vi "NT to Globals & XML.vi"(8 "Array":path[](array[path])) -> ()   [LabVIEW 2020]
uses:
  Utility VIs/NT to XML Number.vi
  Globals/Dashboard_Cal_Globals.vi
panel:
  in  "NT Name Categories":string[](array[string])=["Turret", "Intake", "Magazine", "Flywheel", "FR", "FL", "BL", "BR", "Manual", "Cowl"]
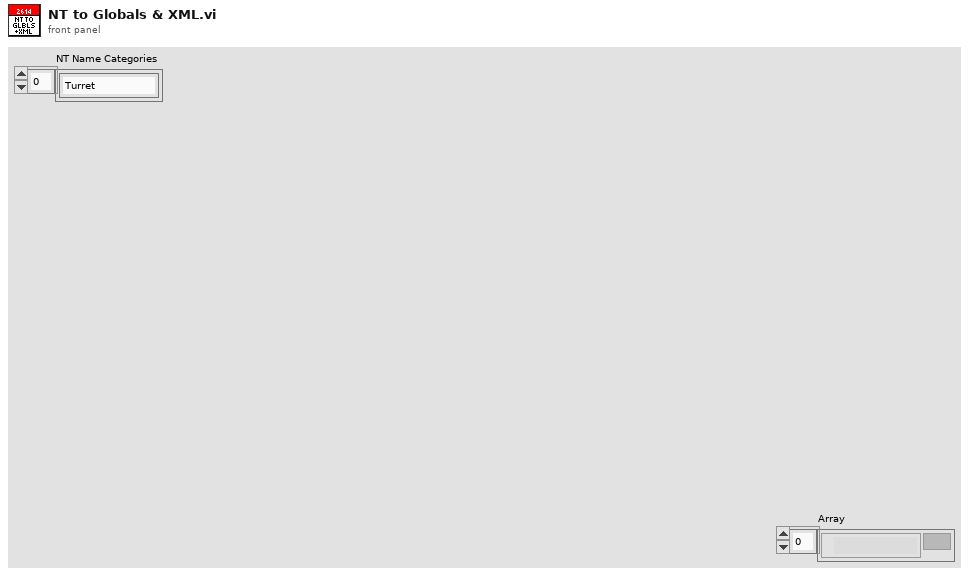
[diagram p1: front panel]
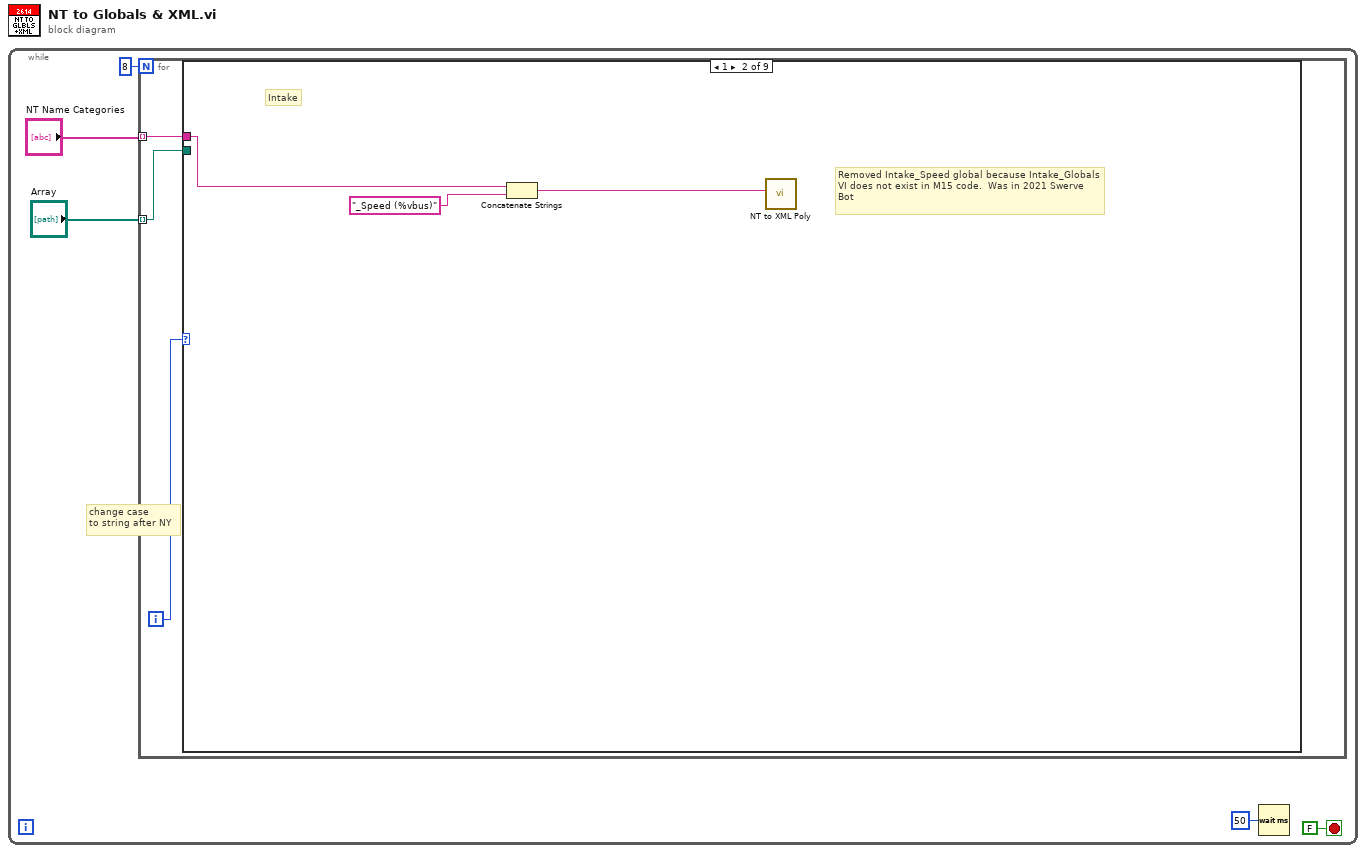
[diagram p0: block diagram]
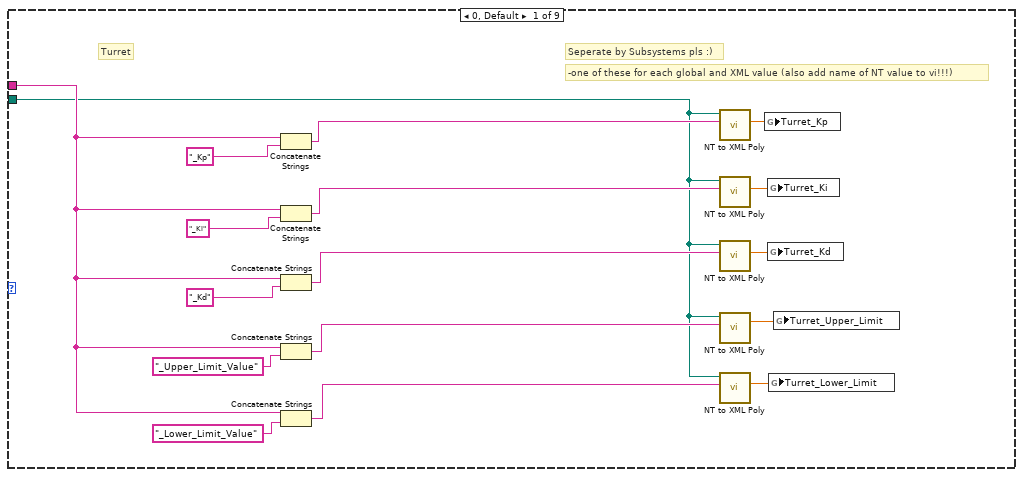
[diagram p2: hidden frame]
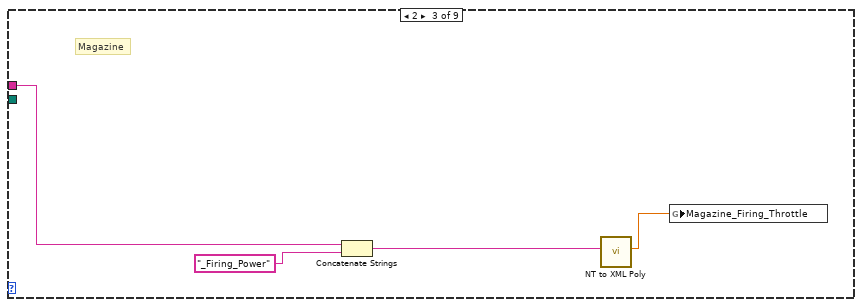
[diagram p3: hidden frame]
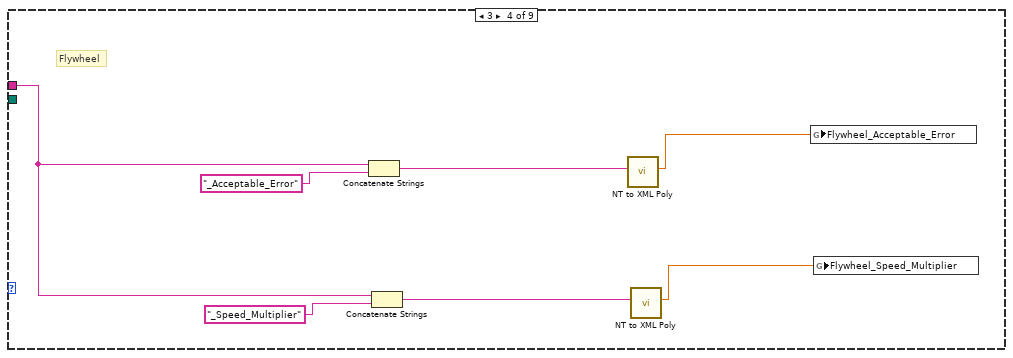
[diagram p4: hidden frame]
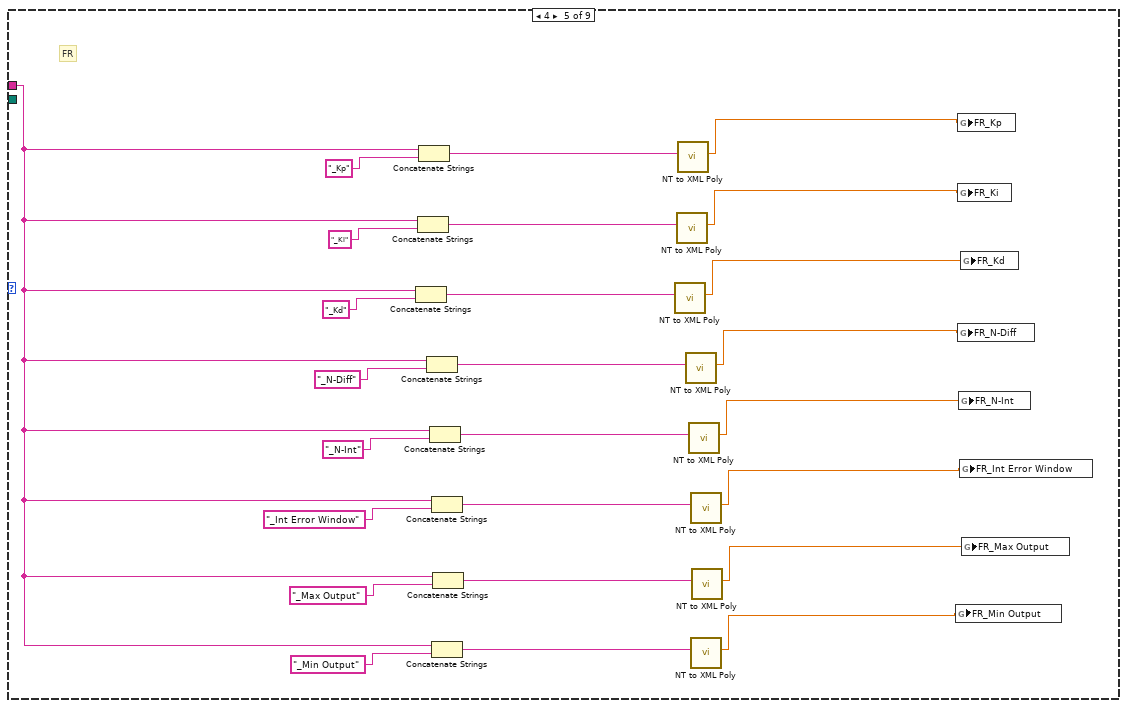
[diagram p5: hidden frame]
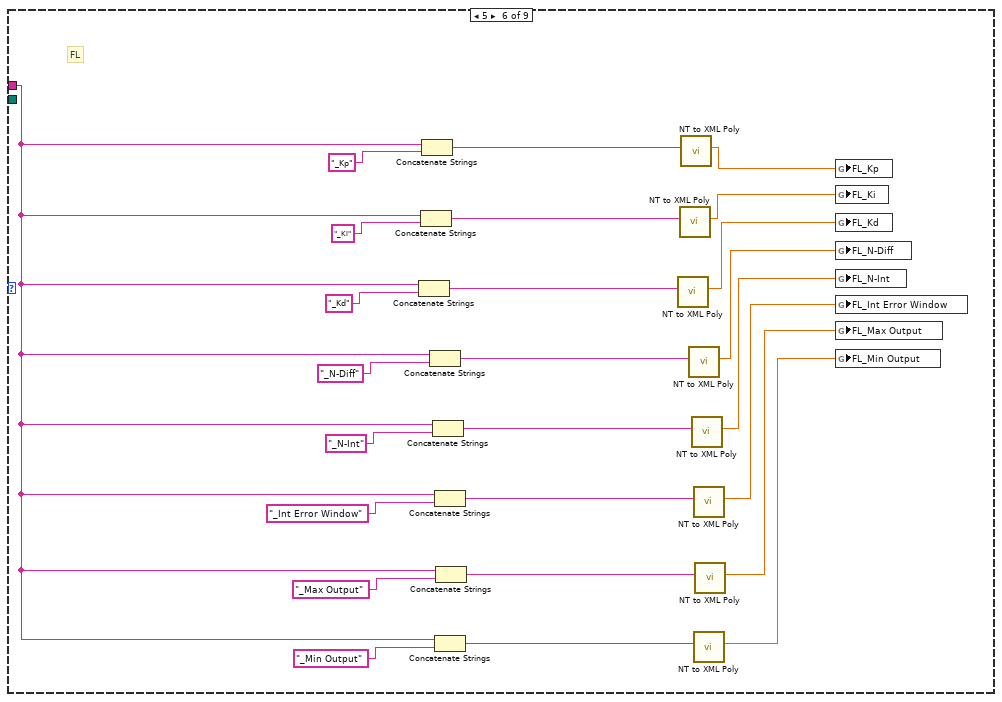
[diagram p6: hidden frame]
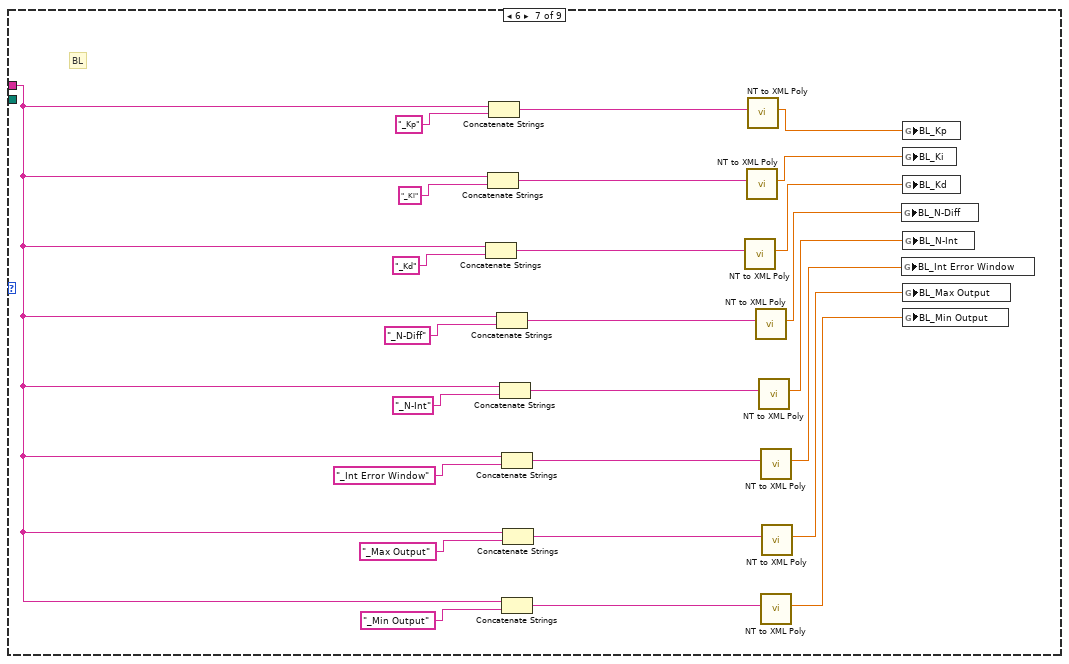
[diagram p7: hidden frame]
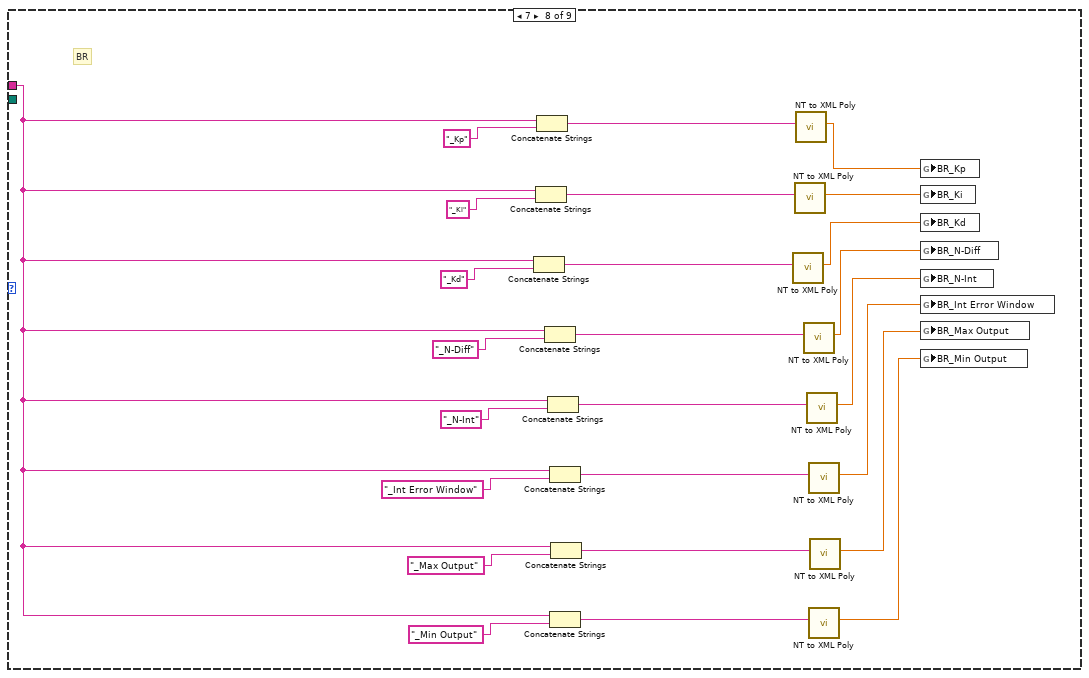
[diagram p8: hidden frame]
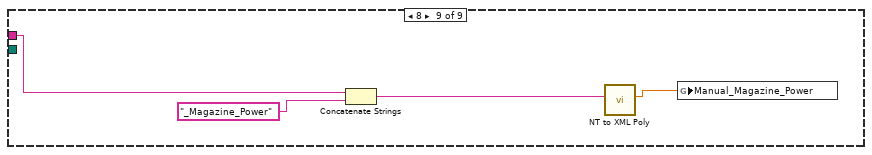
[diagram p9: hidden frame]
diagram:
  n1 = while {
    stop <- FALSE stop-if-true
    # "change case\nto string after NY"
    n2 = for {
      N: 8 -> [_]
      tunnel: "NT Name Categories" -> [w8] mode=indexing
      tunnel: "Array" -> [w7] mode=indexing
      i -> [w6]
      n3 = case shown="1" w6 {
        tunnel: w8 -> [w15 w26 w30 w33 w40 w73 w98 w123 w140]
        tunnel: w7 -> [w9 _ _ _ _ _ _ _ _]
        frame 0, Default {
          # "Turret"
          # "-one of these for each global and XML value (also add name of NT value to vi!!!)"
          # "Seperate by Subsystems pls :)"
          n4 = Concatenate Strings(w15, "_Kp" ("NT Name")) -> (w14:string)
          n5 = Concatenate Strings(w15, "_Ki" ("NT Name")) -> (w13:string)
          n6 = Concatenate Strings(w15, "_Kd" ("NT Name")) -> (w12:string)
          n7 = Concatenate Strings(w15, "_Upper_Limit_Value" ("NT Name")) -> (w11:string)
          n8 = Concatenate Strings(w15, "_Lower_Limit_Value" ("NT Name")) -> (w10:string)
          n9 = call-poly "NT to XML Poly.vi"("NT Name"=w14, "XML File Path"=w9) -> ("Numeric"=w20:dbl)  [unwired: 9 in]
          n10 = call-poly "NT to XML Poly.vi"("NT Name"=w13, "XML File Path"=w9) -> ("Numeric"=w21:dbl)  [unwired: 9 in]
          n11 = call-poly "NT to XML Poly.vi"("NT Name"=w12, "XML File Path"=w9) -> ("Numeric"=w22:dbl)  [unwired: 9 in]
          n12 = call-poly "NT to XML Poly.vi"("NT Name"=w11, "XML File Path"=w9) -> ("Numeric"=w24:dbl)  [unwired: 9 in]
          n13 = call-poly "NT to XML Poly.vi"("NT Name"=w10, "XML File Path"=w9) -> ("Numeric"=w23:dbl)  [unwired: 9 in]
          n14 = global write "Dashboard_Cal_Globals.vi" "Turret_Kp"(w20) -> ()
          n15 = global write "Dashboard_Cal_Globals.vi" "Turret_Ki"(w21) -> ()
          n16 = global write "Dashboard_Cal_Globals.vi" "Turret_Kd"(w22) -> ()
          n17 = global write "Dashboard_Cal_Globals.vi" "Turret_Lower_Limit"(w23) -> ()
          n18 = global write "Dashboard_Cal_Globals.vi" "Turret_Upper_Limit"(w24) -> ()
        }
        frame 1 {
          # "Removed Intake_Speed global because Intake_Globals VI does not exist in M15 code.  Was in 2021 Swerve Bot"
          # "Intake"
          n19 = Concatenate Strings(w26, "_Speed (%vbus)" ("NT Name")) -> (w27:string)
          n20 = call-poly "NT to XML Poly.vi"("NT Name"=w27) -> ()  [unwired: 10 in, 1 out]
        }
        frame 2 {
          # "Magazine"
          n21 = Concatenate Strings(w30, "_Firing_Power" ("NT Name")) -> (w32:string)
          n22 = call-poly "NT to XML Poly.vi"("NT Name"=w32) -> ("Numeric"=w29:dbl)  [unwired: 10 in]
          n23 = global write "Dashboard_Cal_Globals.vi" "Magazine_Firing_Throttle"(w29) -> ()
        }
        frame 3 {
          # "Flywheel"
          n24 = Concatenate Strings(w33, "_Acceptable_Error" ("NT Name")) -> (w39:string)
          n25 = Concatenate Strings(w33, "_Speed_Multiplier" ("NT Name")) -> (w36:string)
          n26 = call-poly "NT to XML Poly.vi"("NT Name"=w39) -> ("Numeric"=w37:dbl)  [unwired: 10 in]
          n27 = call-poly "NT to XML Poly.vi"("NT Name"=w36) -> ("Numeric"=w34:dbl)  [unwired: 10 in]
          n28 = global write "Dashboard_Cal_Globals.vi" "Flywheel_Acceptable_Error"(w37) -> ()
          n29 = global write "Dashboard_Cal_Globals.vi" "Flywheel_Speed_Multiplier"(w34) -> ()
        }
        frame 4 {
          # "FR"
          n30 = Concatenate Strings(w40, "_Kd" ("NT Name")) -> (w60:string)
          n31 = Concatenate Strings(w40, "_Ki" ("NT Name")) -> (w62:string)
          n32 = Concatenate Strings(w40, "_Kp" ("NT Name")) -> (w64:string)
          n33 = Concatenate Strings(w40, "_N-Diff" ("NT Name")) -> (w58:string)
          n34 = Concatenate Strings(w40, "_N-Int" ("NT Name")) -> (w56:string)
          n35 = Concatenate Strings(w40, "_Int Error Window" ("NT Name")) -> (w54:string)
          n36 = Concatenate Strings(w40, "_Min Output" ("NT Name")) -> (w50:string)
          n37 = Concatenate Strings(w40, "_Max Output" ("NT Name")) -> (w52:string)
          n38 = call-poly "NT to XML Poly.vi"("NT Name"=w60) -> ("Numeric"=w46:dbl)  [unwired: 10 in]
          n39 = call-poly "NT to XML Poly.vi"("NT Name"=w62) -> ("Numeric"=w47:dbl)  [unwired: 10 in]
          n40 = call-poly "NT to XML Poly.vi"("NT Name"=w64) -> ("Numeric"=w48:dbl)  [unwired: 10 in]
          n41 = call-poly "NT to XML Poly.vi"("NT Name"=w58) -> ("Numeric"=w45:dbl)  [unwired: 10 in]
          n42 = call-poly "NT to XML Poly.vi"("NT Name"=w56) -> ("Numeric"=w44:dbl)  [unwired: 10 in]
          n43 = call-poly "NT to XML Poly.vi"("NT Name"=w54) -> ("Numeric"=w43:dbl)  [unwired: 10 in]
          n44 = call-poly "NT to XML Poly.vi"("NT Name"=w50) -> ("Numeric"=w41:dbl)  [unwired: 10 in]
          n45 = call-poly "NT to XML Poly.vi"("NT Name"=w52) -> ("Numeric"=w42:dbl)  [unwired: 10 in]
          n46 = global write "Dashboard_Cal_Globals.vi" "FR_Min Output"(w41) -> ()
          n47 = global write "Dashboard_Cal_Globals.vi" "FR_Kp"(w48) -> ()
          n48 = global write "Dashboard_Cal_Globals.vi" "FR_Ki"(w47) -> ()
          n49 = global write "Dashboard_Cal_Globals.vi" "FR_N-Diff"(w45) -> ()
          n50 = global write "Dashboard_Cal_Globals.vi" "FR_N-Int"(w44) -> ()
          n51 = global write "Dashboard_Cal_Globals.vi" "FR_Int Error Window"(w43) -> ()
          n52 = global write "Dashboard_Cal_Globals.vi" "FR_Kd"(w46) -> ()
          n53 = global write "Dashboard_Cal_Globals.vi" "FR_Max Output"(w42) -> ()
        }
        frame 5 {
          # "FL"
          n54 = Concatenate Strings(w73, "_Kd" ("NT Name")) -> (w85:string)
          n55 = Concatenate Strings(w73, "_Ki" ("NT Name")) -> (w87:string)
          n56 = Concatenate Strings(w73, "_Kp" ("NT Name")) -> (w89:string)
          n57 = Concatenate Strings(w73, "_N-Diff" ("NT Name")) -> (w83:string)
          n58 = Concatenate Strings(w73, "_N-Int" ("NT Name")) -> (w81:string)
          n59 = Concatenate Strings(w73, "_Int Error Window" ("NT Name")) -> (w79:string)
          n60 = Concatenate Strings(w73, "_Min Output" ("NT Name")) -> (w75:string)
          n61 = Concatenate Strings(w73, "_Max Output" ("NT Name")) -> (w77:string)
          n62 = call-poly "NT to XML Poly.vi"("NT Name"=w85) -> ("Numeric"=w70:dbl)  [unwired: 10 in]
          n63 = call-poly "NT to XML Poly.vi"("NT Name"=w87) -> ("Numeric"=w71:dbl)  [unwired: 10 in]
          n64 = call-poly "NT to XML Poly.vi"("NT Name"=w89) -> ("Numeric"=w72:dbl)  [unwired: 10 in]
          n65 = call-poly "NT to XML Poly.vi"("NT Name"=w83) -> ("Numeric"=w69:dbl)  [unwired: 10 in]
          n66 = call-poly "NT to XML Poly.vi"("NT Name"=w81) -> ("Numeric"=w68:dbl)  [unwired: 10 in]
          n67 = call-poly "NT to XML Poly.vi"("NT Name"=w79) -> ("Numeric"=w67:dbl)  [unwired: 10 in]
          n68 = call-poly "NT to XML Poly.vi"("NT Name"=w75) -> ("Numeric"=w65:dbl)  [unwired: 10 in]
          n69 = call-poly "NT to XML Poly.vi"("NT Name"=w77) -> ("Numeric"=w66:dbl)  [unwired: 10 in]
          n70 = global write "Dashboard_Cal_Globals.vi" "FL_Kp"(w72) -> ()
          n71 = global write "Dashboard_Cal_Globals.vi" "FL_Ki"(w71) -> ()
          n72 = global write "Dashboard_Cal_Globals.vi" "FL_Kd"(w70) -> ()
          n73 = global write "Dashboard_Cal_Globals.vi" "FL_N-Diff"(w69) -> ()
          n74 = global write "Dashboard_Cal_Globals.vi" "FL_N-Int"(w68) -> ()
          n75 = global write "Dashboard_Cal_Globals.vi" "FL_Int Error Window"(w67) -> ()
          n76 = global write "Dashboard_Cal_Globals.vi" "FL_Max Output"(w66) -> ()
          n77 = global write "Dashboard_Cal_Globals.vi" "FL_Min Output"(w65) -> ()
        }
        frame 6 {
          # "BL"
          n78 = Concatenate Strings(w98, "_Kd" ("NT Name")) -> (w110:string)
          n79 = Concatenate Strings(w98, "_Ki" ("NT Name")) -> (w112:string)
          n80 = Concatenate Strings(w98, "_Kp" ("NT Name")) -> (w114:string)
          n81 = Concatenate Strings(w98, "_N-Diff" ("NT Name")) -> (w108:string)
          n82 = Concatenate Strings(w98, "_N-Int" ("NT Name")) -> (w106:string)
          n83 = Concatenate Strings(w98, "_Int Error Window" ("NT Name")) -> (w104:string)
          n84 = Concatenate Strings(w98, "_Min Output" ("NT Name")) -> (w100:string)
          n85 = Concatenate Strings(w98, "_Max Output" ("NT Name")) -> (w102:string)
          n86 = call-poly "NT to XML Poly.vi"("NT Name"=w110) -> ("Numeric"=w95:dbl)  [unwired: 10 in]
          n87 = call-poly "NT to XML Poly.vi"("NT Name"=w112) -> ("Numeric"=w96:dbl)  [unwired: 10 in]
          n88 = call-poly "NT to XML Poly.vi"("NT Name"=w114) -> ("Numeric"=w97:dbl)  [unwired: 10 in]
          n89 = call-poly "NT to XML Poly.vi"("NT Name"=w108) -> ("Numeric"=w94:dbl)  [unwired: 10 in]
          n90 = call-poly "NT to XML Poly.vi"("NT Name"=w106) -> ("Numeric"=w93:dbl)  [unwired: 10 in]
          n91 = call-poly "NT to XML Poly.vi"("NT Name"=w104) -> ("Numeric"=w92:dbl)  [unwired: 10 in]
          n92 = call-poly "NT to XML Poly.vi"("NT Name"=w100) -> ("Numeric"=w90:dbl)  [unwired: 10 in]
          n93 = call-poly "NT to XML Poly.vi"("NT Name"=w102) -> ("Numeric"=w91:dbl)  [unwired: 10 in]
          n94 = global write "Dashboard_Cal_Globals.vi" "BL_N-Diff"(w94) -> ()
          n95 = global write "Dashboard_Cal_Globals.vi" "BL_Int Error Window"(w92) -> ()
          n96 = global write "Dashboard_Cal_Globals.vi" "BL_Kp"(w97) -> ()
          n97 = global write "Dashboard_Cal_Globals.vi" "BL_Ki"(w96) -> ()
          n98 = global write "Dashboard_Cal_Globals.vi" "BL_Kd"(w95) -> ()
          n99 = global write "Dashboard_Cal_Globals.vi" "BL_N-Int"(w93) -> ()
          n100 = global write "Dashboard_Cal_Globals.vi" "BL_Max Output"(w91) -> ()
          n101 = global write "Dashboard_Cal_Globals.vi" "BL_Min Output"(w90) -> ()
        }
        frame 7 {
          # "BR"
          n102 = Concatenate Strings(w123, "_Kd" ("NT Name")) -> (w134:string)
          n103 = Concatenate Strings(w123, "_Ki" ("NT Name")) -> (w133:string)
          n104 = Concatenate Strings(w123, "_Kp" ("NT Name")) -> (w132:string)
          n105 = Concatenate Strings(w123, "_N-Diff" ("NT Name")) -> (w135:string)
          n106 = Concatenate Strings(w123, "_N-Int" ("NT Name")) -> (w136:string)
          n107 = Concatenate Strings(w123, "_Int Error Window" ("NT Name")) -> (w137:string)
          n108 = Concatenate Strings(w123, "_Min Output" ("NT Name")) -> (w139:string)
          n109 = Concatenate Strings(w123, "_Max Output" ("NT Name")) -> (w138:string)
          n110 = call-poly "NT to XML Poly.vi"("NT Name"=w134) -> ("Numeric"=w120:dbl)  [unwired: 10 in]
          n111 = call-poly "NT to XML Poly.vi"("NT Name"=w133) -> ("Numeric"=w121:dbl)  [unwired: 10 in]
          n112 = call-poly "NT to XML Poly.vi"("NT Name"=w132) -> ("Numeric"=w122:dbl)  [unwired: 10 in]
          n113 = call-poly "NT to XML Poly.vi"("NT Name"=w135) -> ("Numeric"=w119:dbl)  [unwired: 10 in]
          n114 = call-poly "NT to XML Poly.vi"("NT Name"=w136) -> ("Numeric"=w118:dbl)  [unwired: 10 in]
          n115 = call-poly "NT to XML Poly.vi"("NT Name"=w137) -> ("Numeric"=w117:dbl)  [unwired: 10 in]
          n116 = call-poly "NT to XML Poly.vi"("NT Name"=w139) -> ("Numeric"=w115:dbl)  [unwired: 10 in]
          n117 = call-poly "NT to XML Poly.vi"("NT Name"=w138) -> ("Numeric"=w116:dbl)  [unwired: 10 in]
          n118 = global write "Dashboard_Cal_Globals.vi" "BR_Kp"(w122) -> ()
          n119 = global write "Dashboard_Cal_Globals.vi" "BR_Ki"(w121) -> ()
          n120 = global write "Dashboard_Cal_Globals.vi" "BR_Kd"(w120) -> ()
          n121 = global write "Dashboard_Cal_Globals.vi" "BR_N-Diff"(w119) -> ()
          n122 = global write "Dashboard_Cal_Globals.vi" "BR_N-Int"(w118) -> ()
          n123 = global write "Dashboard_Cal_Globals.vi" "BR_Int Error Window"(w117) -> ()
          n124 = global write "Dashboard_Cal_Globals.vi" "BR_Max Output"(w116) -> ()
          n125 = global write "Dashboard_Cal_Globals.vi" "BR_Min Output"(w115) -> ()
        }
        frame 8 {
          n126 = Concatenate Strings(w140, "_Magazine_Power" ("NT Name")) -> (w142:string)
          n127 = call-poly "NT to XML Poly.vi"("NT Name"=w142) -> ("Numeric"=w143:dbl)  [unwired: 10 in]
          n128 = global write "Dashboard_Cal_Globals.vi" "Manual_Magazine_Power"(w143) -> ()
        }
      }
    }
    n129 = Wait (ms)(milliseconds to wait=u32 50) -> ()  [unwired: 1 out]
  }
